vi "Filter Rules - v1.0.vi"(11 "Rules-v1":T1) -> (3 "GlobalLogFilter out":refnum<class "GlobalLogFilter.lvclass">)   [LabVIEW 2017]
uses:
  GlobalLogFilter.lvclass
  CSM GlobalLog Filter Rules - v1.0.ctl
  _Support/Typedef/_CSM_GlobalLog_MSG_TYPE.ctl
  Communicable State Machine.lvlib
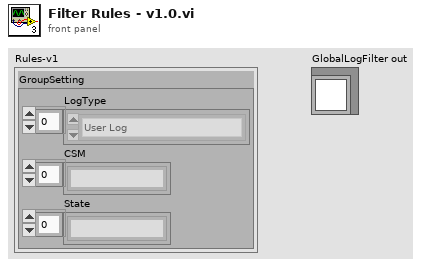
[diagram p1: front panel]
types:
  T1 = typedef "CSM GlobalLog Filter Rules - v1.0.ctl" = cluster{"GroupSetting":cluster{"LogType":T2[], "CSM":string[], "State":string[]}}
  T2 = typedef "Communicable State Machine.lvlib/_CSM_GlobalLog_MSG_TYPE.ctl" = enum16{"User Log", "State Change", "Status", "Interrupt", "Register", "Unregister", "Error Log", "Module Created", "Module Destroyed"}
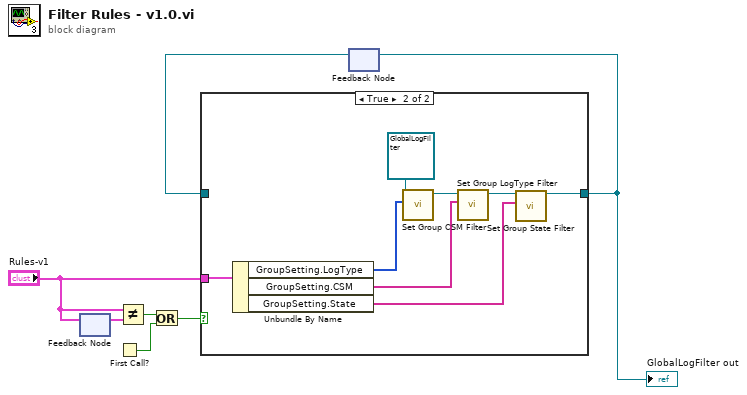
[diagram p0: block diagram]
diagram:
  n1 = feedback #1() -> (w2:T1)  [unwired: 1 in]
  n2 = feedback-in #1("Rules-v1") -> ()
  n3 = First Call?() -> (First Call?: T/F=w4:bool)
  n4 = Not Equal?(x="Rules-v1", y=w2) -> (x != y?=w3:bool)
  n5 = Or(x=w3, y=w4) -> (x .or. y?=w5:bool)
  n6 = feedback #2() -> (w7:refnum<class "GlobalLogFilter.lvclass">)  [unwired: 1 in]
  n7 = case shown="True" w5 {
    tunnel: [w8 w10] -> w6
    tunnel: "Rules-v1" -> [_ w12]
    tunnel: w7 -> [w8 _]
    frame False {
    }
    frame True {
      n8 = Unbundle By Name(w12) -> ("GroupSetting.LogType"=w14:T2[], "GroupSetting.CSM"=w13:string[], "GroupSetting.State"=w9:string[])
      n9 = call "Set Group CSM Filter.vi"("Group:LogType"=w14, "GlobalLogFilter in"=refnum<class "GlobalLogFilter.lvclass"> refnum ("GlobalLogFilter.lvclass")) -> ("GlobalLogFilter out"=w15:refnum<class "GlobalLogFilter.lvclass">)  [unwired: 8 in, 1 out]
      n10 = call "Set Group LogType Filter.vi"("Group:CSM"=w13, "GlobalLogFilter in"=w15) -> ("GlobalLogFilter out"=w11:refnum<class "GlobalLogFilter.lvclass">)  [unwired: 8 in, 1 out]
      n11 = call "Set Group State Filter.vi"("Group:State"=w9, "GlobalLogFilter in"=w11) -> ("GlobalLogFilter out"=w10:refnum<class "GlobalLogFilter.lvclass">)  [unwired: 8 in, 1 out]
    }
  }
  "GlobalLogFilter out" <- w6
  n12 = feedback-in #2(w6) -> ()
